vi "Get App Name.vi"(8 "错误输入（无错误）":errorcluster) -> (0 "错误输出":errorcluster, 3 "应用程序:名称":string)   [LabVIEW 2012, in "Application.lvlib"]
uses:
  Application.lvlib
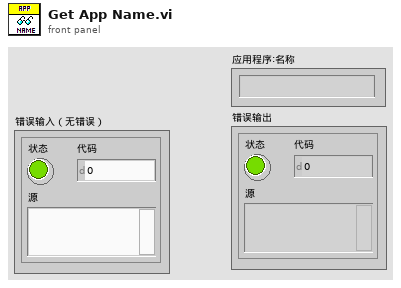
[diagram p1: front panel]
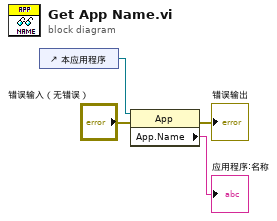
[diagram p0: block diagram]
diagram:
  n1 = control-ref of="本应用程序"() -> (w4:refnum<vi>)
  n2 = property class="App"(reference=w4, error in="错误输入（无错误）") -> (error out=→"错误输出":errorcluster, "App.Name"=→"应用程序:名称":string)  [unwired: 1 out]
